vi "Verify.Caraya.vi"(8 "error in (no error)":errorcluster, 11 "Test Data":string) -> (0 "error out":errorcluster)   [LabVIEW 2020]
uses:
  <vilib>/addons/_JKI Toolkits/Caraya/classes/Assert/Assert True.vi
  <vilib>/SAS/Approval Tests/lib_Approval Tests.lvlib
  <vilib>/addons/_JKI Toolkits/Caraya/classes/Assert/Assert.lvclass
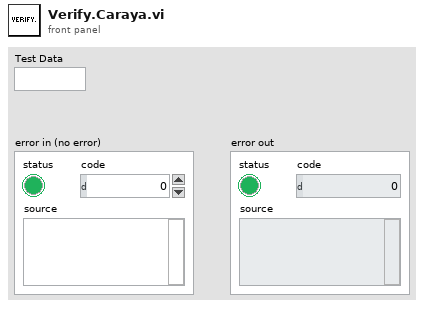
[diagram p1: front panel]
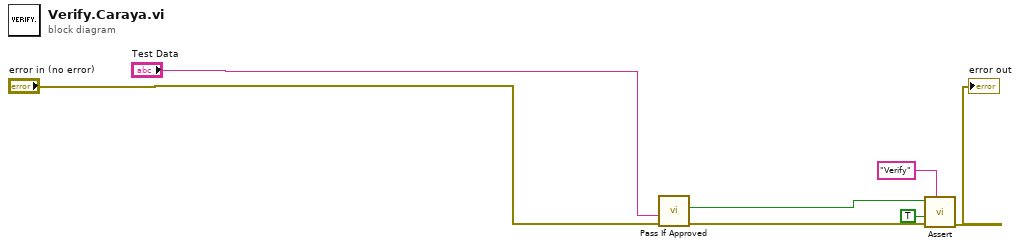
[diagram p0: block diagram]
diagram:
  n1 = call <vilib>:"Pass If Approved.vi"("error in"="error in (no error)", "Test Data"="Test Data") -> ("error out"=w2:errorcluster, "Passed?"=w4:bool)  [unwired: 7 in, 1 out]
  n2 = call-poly <vilib>:"Assert.vi"("Label"="Verify", "error in (no error)"=w2, "Register with caller test (F)"=TRUE, "True?"=w4) -> ("error out"=→"error out":errorcluster)  [unwired: 6 in, 1 out]
